vi "Append Time String.vi"(4 "enable (T)":bool=TRUE, 5 "error in":errorcluster, 8 "string in":string="User error message.") -> (0 "error out":errorcluster {"code" format="%.0x"}, 3 "string out":string)   [LabVIEW 2020]
doc: "This function appends the current time ( at HR:MN AM/PM format) to a string. If the string has a trailing period, it will be replaced with a period after the appended time."
panel:
  # "Trim period, append \" at \", current time AM/PM, period.\n\nExample \"at 10:21 AM.\""
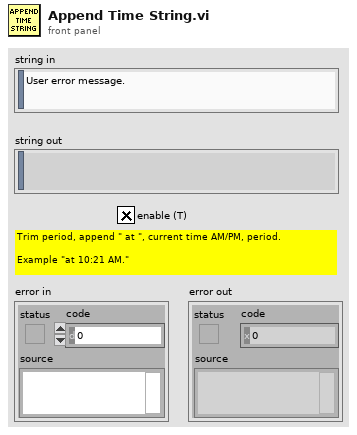
[diagram p1: front panel]
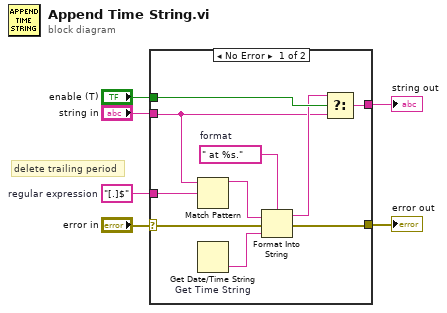
[diagram p0: block diagram]
diagram:
  w1 = "[.]$"  # regular expression
  # "delete trailing period"
  n1 = case shown="No Error" "error in" {
    selector: "error in" -> [w10 w17]
    tunnel: [w11 w17] -> w6
    tunnel: "enable (T)" -> [w14 _]
    tunnel: "string in" -> [w8 w18]
    tunnel: [w9 w18] -> w2
    tunnel: w1 -> [w7 _]
    frame No Error {
      w16 = " at %s."  # format
      n2 = Match Pattern(string=w8, regular expression=w7) -> (before substring=w12:string)  [unwired: 1 in, 3 out]
      n3 = Get Date/Time String "Get Time String"() -> (time string=w15:string)  [unwired: 3 in, 1 out]
      n4 = Format Into String(format string=w16, initial string=w12, error in=w10, w15) -> (resulting string=w13:string, error out=w11:errorcluster)
      n5 = Select(t=w13, s=w14, f=w8) -> (s? t:f=w9:string)
    }
    frame Error {
    }
  }
  "error out" <- w6
  "string out" <- w2
